vi "GetChannelData.vi"(0 "SmartScope in":refnum<k24>, 1 "LatestDataPackage":refnum<k24>, 2 "AnalogChannel":refnum<k24>) -> (3 "SmartScope out":refnum<k24>, 4 "Waveform Graph":dbl[](array[numeric]), 5 "ViewportBegin":dbl, 6 "ViewportEnd":dbl)   [LabVIEW 2019]
uses:
  C:/Program Files (x86)/LabNation/SmartScope/DeviceInterface.dll
  Program Files (x86)/LabNation/SmartScope/DeviceInterface.dll
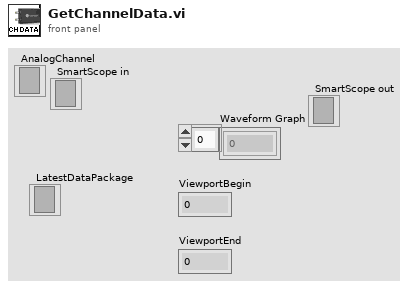
[diagram p1: front panel]
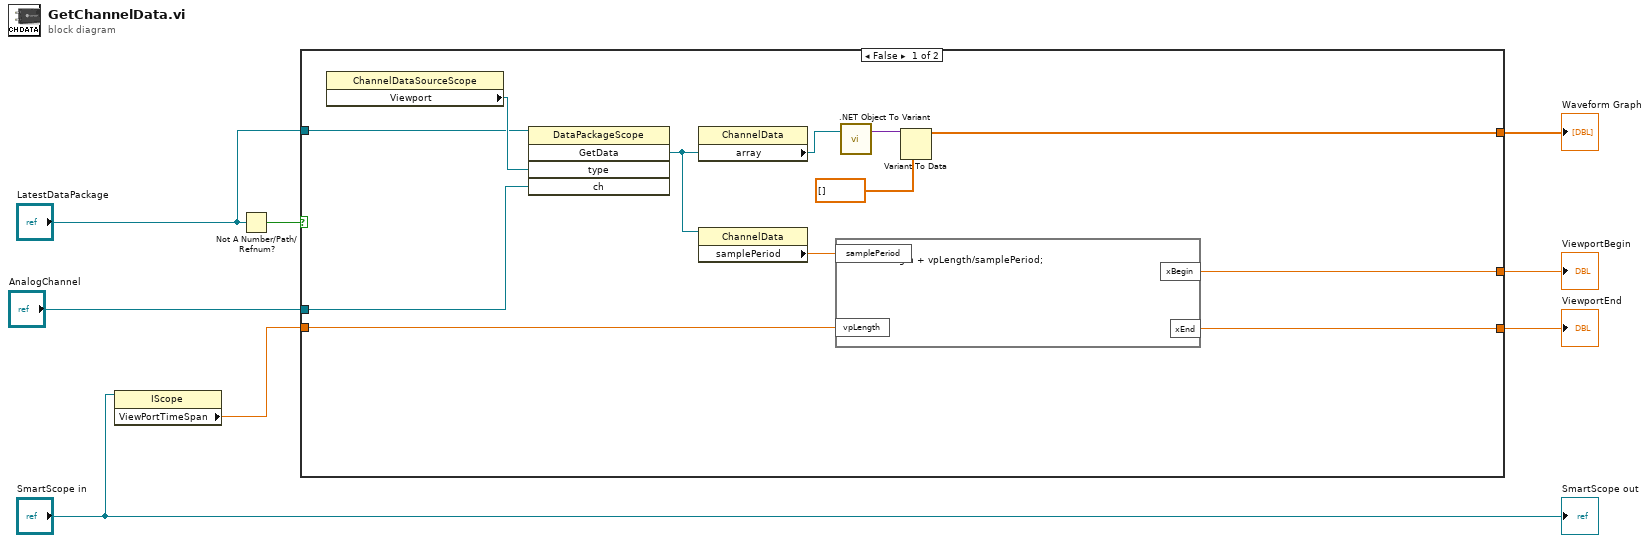
[diagram p0: block diagram]
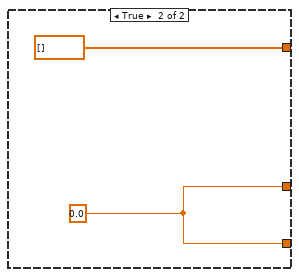
[diagram p2: hidden frame]
diagram:
  n1 = property class="IScope"(reference="SmartScope in") -> ("ViewPortTimeSpan"=w2:dbl)  [unwired: 1 in, 2 out]
  n2 = Not A Number/Path/Refnum?(number/path/refnum="LatestDataPackage") -> (NaN/Path/Refnum?=w7:bool)
  n3 = case shown="False" w7 {
    tunnel: "LatestDataPackage" -> [w17 _]
    tunnel: w2 -> [w15 _]
    tunnel: [w14 dbl[] [] ("Waveform Graph")] -> w6
    tunnel: [w13 w21] -> w4
    tunnel: [w12 w21] -> w5
    tunnel: "AnalogChannel" -> [w11 _]
    frame False {
      n4 = property class="ChannelDataSourceScope"() -> ("Viewport"=w20:refnum<k24>)  [unwired: 2 in, 2 out]
      n5 = invoke class="DataPackageScope" method="GetData"(reference=w17, "type"=w20, "ch"=w11) -> ("GetData"=w18:refnum<k24>)  [unwired: 2 in, 4 out]
      n6 = property class="ChannelData"(reference=w18) -> ("array"=w10:refnum<k24>)  [unwired: 1 in, 2 out]
      n7 = property class="ChannelData"(reference=w18) -> ("samplePeriod"=w16:dbl)  [unwired: 1 in, 2 out]
      n8 = formula code="xBegin = 0;\nxEnd = xBegin + vpLength/samplePeriod;"("samplePeriod"=w16, "vpLength"=w15) -> ("xBegin"=w13:dbl, "xEnd"=w12:dbl)
      n9 = call <vilib>:".NET Object To Variant.vi"(".NET object"=w10) -> ("variant"=w9:variant)  [unwired: 1 in, 1 out]
      n10 = Variant To Data(type=dbl[] [] ("Waveform Graph"), Variant=w9) -> (data=w14:dbl[])  [unwired: 1 in, 1 out]
    }
    frame True {
      w21 = 0.0 ("xBegin")
    }
  }
  "Waveform Graph" <- w6
  "ViewportEnd" <- w5
  "ViewportBegin" <- w4
  "SmartScope out" <- "SmartScope in"
